vi "GLdrv_COMMON_IDN.vi"(0 "Connection ID":T1, 11 "error in (no error)":errorcluster) -> (4 "Connection ID Out":T1, 6 "IDN out":string, 15 "error out":errorcluster)   [LabVIEW 2017, in "GL860_Driver.lvlib"]
doc: "IDNの参照"
uses:
  GL860_Driver.lvlib
  ConnectionID.ctl
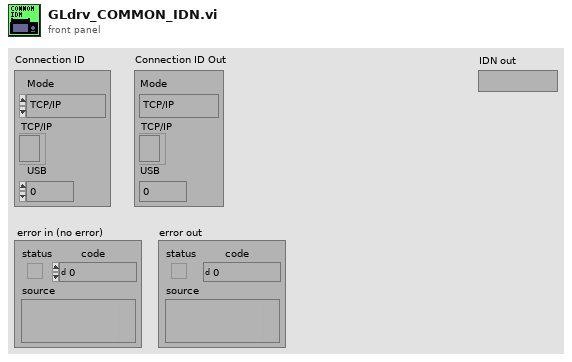
[diagram p1: front panel]
types:
  T1 = typedef "ConnectionID.ctl" = cluster{"Mode":enum16{"TCP/IP", "USB"}, "TCP/IP":refnum<k5>, "USB":i32}
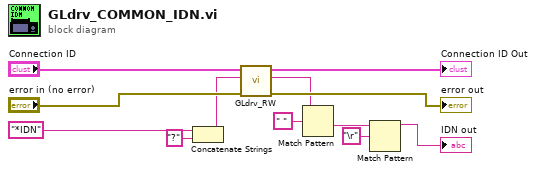
[diagram p0: block diagram]
diagram:
  n1 = Concatenate Strings("*IDN" ("Command"), "?" ("string")) -> (w3:string)
  n2 = call "GLdrv_RW.vi"("error in (no error)"="error in (no error)", "data in"=w3, "Connection ID"="Connection ID") -> ("error out"=→"error out":errorcluster, "data out"=w2:string, "Connection ID Out"=→"Connection ID Out":T1)  [unwired: 4 in, 2 out]
  n3 = Match Pattern(string=w2, regular expression=" " ("search string/char (-)")) -> (after substring=w5:string)  [unwired: 4 out]
  n4 = Match Pattern(string=w5, regular expression="\r") -> (before substring=→"IDN out":string)  [unwired: 4 out]
